vi "Forward Error to Caller.vi"(8 "error in":errorcluster, 11 "Actor":refnum<class "_Parent Actor Template.lvclass">) -> (0 "error out":errorcluster, 2 "Shutdown":bool, 3 "Actor out":refnum<class "_Parent Actor Template.lvclass">)   [LabVIEW 2016, in "_Parent Actor Template.lvlib" / "_Parent Actor Template.lvclass"]
doc: "Forwards any unrecognized errors to the calling actor for handling.\n\nReturns shutdown boolean TRUE for the following errors: 43, 1608, and 1556.\n\n43, 1608:\nStop on Normal Stop and Emergency Stop errors.\n\n1556:\nAlso stop if calling Actor has stopped. (invalid enqueuer error)"
uses:
  _Parent Actor Template.lvclass
  C:/Program Files (x86)/National Instruments/LabVIEW 2016/vi.lib/ActorFramework/Actor/Actor.lvclass
  <vilib>/ActorFramework/Actor/Actor.lvclass/Actor.ctl
  <vilib>/ActorFramework/Actor/Actor.lvclass
  _Parent Actor Template Messages/Receive Error Msg/Receive Error Msg.lvclass
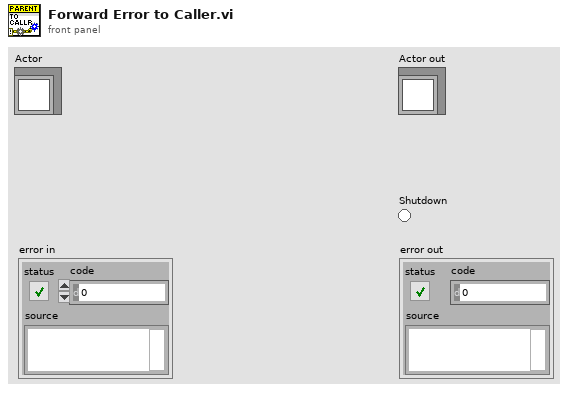
[diagram p1: front panel]
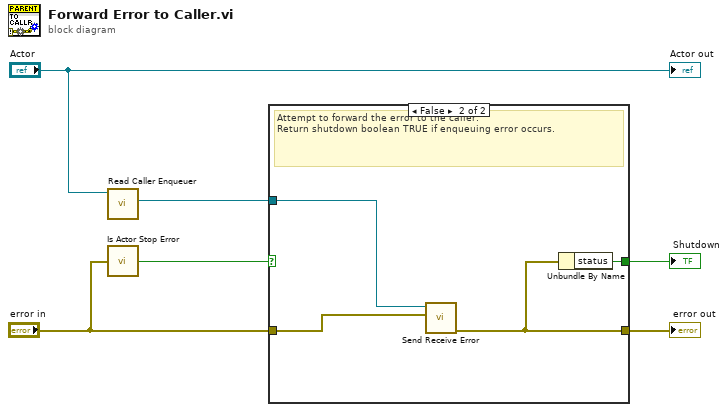
[diagram p0: block diagram]
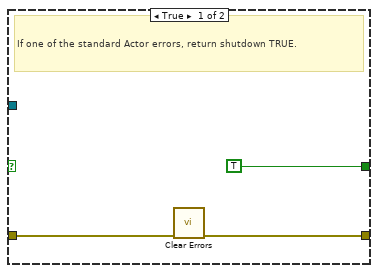
[diagram p2: hidden frame]
diagram:
  n1 = call <vilib>:"Read Caller Enqueuer.vi"("Actor"="Actor") -> ("Caller Enqueuer"=w2:refnum<class "Message Enqueuer.lvclass">)  [unwired: 10 in]
  n2 = call "Is Actor Stop Error.vi"("error in"="error in") -> ("Stop Error"=w1:bool)
  n3 = case shown="False" w1 {
    tunnel: "error in" -> [w8 w11]
    tunnel: [w7 w10] -> w4
    tunnel: [TRUE ("Shutdown") w13] -> w5
    tunnel: w2 -> [_ w12]
    frame True {
      # "If one of the standard Actor errors, return shutdown TRUE."
      n4 = call <vilib>:"Clear Errors.vi"("error in (no error)"=w8) -> ("error out"=w7:errorcluster)  [unwired: 5 in, 1 out]
    }
    frame False {
      # "Attempt to forward the error to the caller.\nReturn shutdown boolean TRUE if enqueuing error occurs."
      n5 = call "Send Receive Error.vi"("Receive Error"=w11, "Message Enqueuer in"=w12) -> ("error out"=w10:errorcluster)  [unwired: 8 in, 1 out]
      n6 = Unbundle By Name(w10) -> ("status"=w13:bool)
    }
  }
  "Shutdown" <- w5
  "error out" <- w4
  "Actor out" <- "Actor"
